vi "LaserConfigure.vi"(2 "error in":errorcluster, 5 "Laser Power":i32, 7 "SeedLaserPower":T1) -> ()   [LabVIEW 2011]
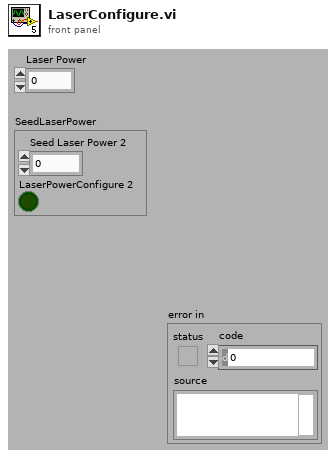
[diagram p1: front panel]
types:
  T1 = cluster{"Seed Laser Power 2":i8, "LaserPowerConfigure 2":bool}
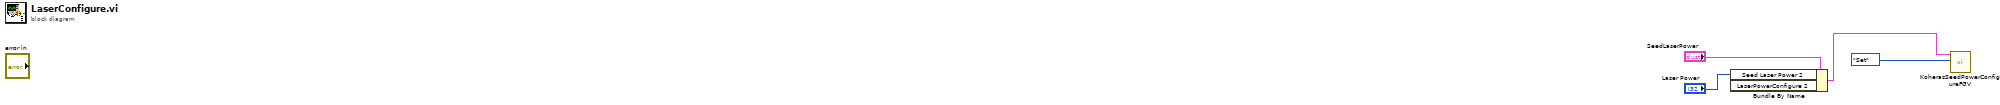
[diagram p0: block diagram]
diagram:
  n1 = Bundle By Name(cluster="SeedLaserPower", "Seed Laser Power 2"="Laser Power") -> (w3:T1)  [unwired: 1 in]
  n2 = call "KoherasSeedPowerConfigureFGV.vi"("Set_Get"=enum16{"Set", "Get"}."Set", "SeedLaserPower"=w3) -> ()  [unwired: 8 in, 2 out]
